vi "GetAllQueueStatus.vi"(8 "error in":errorcluster, 11 "queues in":refnum<class "CLM_PriorityLocalMessage.lvclass">) -> (0 "error out":errorcluster, 1 "max queue size[]":i32[](array[numeric]), 2 "# elements in queue[]":i32[](array[numeric]), 3 "queues out":refnum<class "CLM_PriorityLocalMessage.lvclass">, 4 "# pending remove[]":i32[](array[numeric]), 5 "priority[]":i32[](array[numeric]), 6 "# pending insert[]":i32[](array[numeric]))   [LabVIEW 2013, in "CLM_PriorityLocalMessage.lvclass"]
uses:
  CLM_PriorityLocalMessage.lvclass
  CLM_PriorityLocalMessage.lvclass/CLM_PriorityLocalMessage.ctl
  LocalMessage_Queue/CLM_LocalMessage_Queue.lvclass/CLM_LocalMessage_Queue.ctl
  LocalMessage_Queue/CLM_LocalMessage_Queue.lvclass
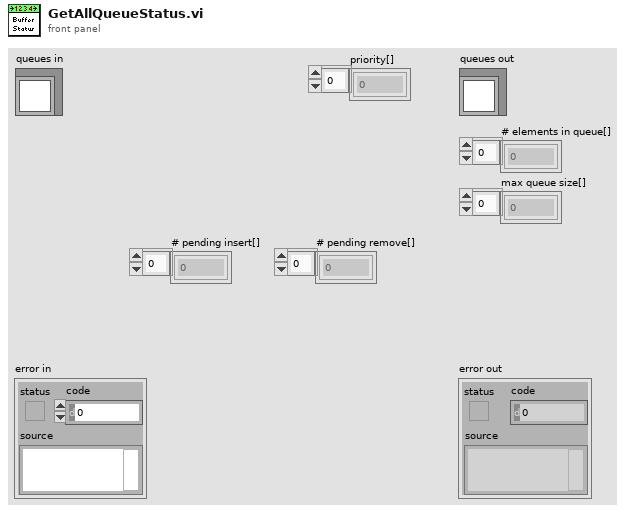
[diagram p1: front panel]
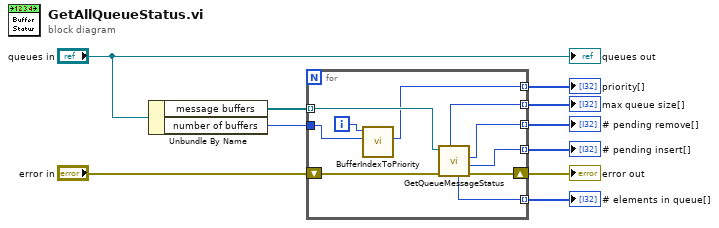
[diagram p0: block diagram]
diagram:
  n1 = Unbundle By Name("queues in") -> ("message buffers"=w9:refnum<class "CLM_LocalMessage_Queue.lvclass">[], "number of buffers"=w8:i32)
  n2 = for {
    tunnel: w9 -> [w20] mode=indexing
    shift-right: [w19] -> w2
    shift-left: "error in" -> [w18]
    tunnel: w8 -> [w17]
    tunnel: [w15] -> w7 mode=indexing
    tunnel: [w14] -> w6 mode=indexing
    tunnel: [w13] -> w5 mode=indexing
    tunnel: [w12] -> w4 mode=indexing
    tunnel: [w11] -> w3 mode=indexing
    i -> [w16]
    n3 = call "BufferIndexToPriority.vi"("number of buffers"=w17, "buffer index"=w16) -> ("priority"=w15:i32)  [unwired: 6 in, 3 out]
    n4 = call "GetQueueMessageStatus.vi"("error in"=w18, "message ref in"=w20) -> ("error out"=w19:errorcluster, "# pending insert"=w12:i32, "# pending remove"=w13:i32, "# elements in queue"=w11:i32, "max queue size"=w14:i32)  [unwired: 2 in, 3 out]
  }
  "error out" <- w2
  "priority[]" <- w7
  "max queue size[]" <- w6
  "# pending remove[]" <- w5
  "# pending insert[]" <- w4
  "# elements in queue[]" <- w3
  "queues out" <- "queues in"
